vi "Read Action settings.vi"(8 "error in (no error)":errorcluster, 11 "Motor in":refnum<class "Motor.lvclass">) -> (0 "error out":errorcluster, 2 "Action settings":T1, 3 "Motor out":refnum<class "Motor.lvclass">)   [LabVIEW 2013, in "PowderDeposition.lvlib" / "Motor.lvclass"]
uses:
  Motor.lvclass
  Action-settings.ctl
  Motor.lvclass/Motor.ctl
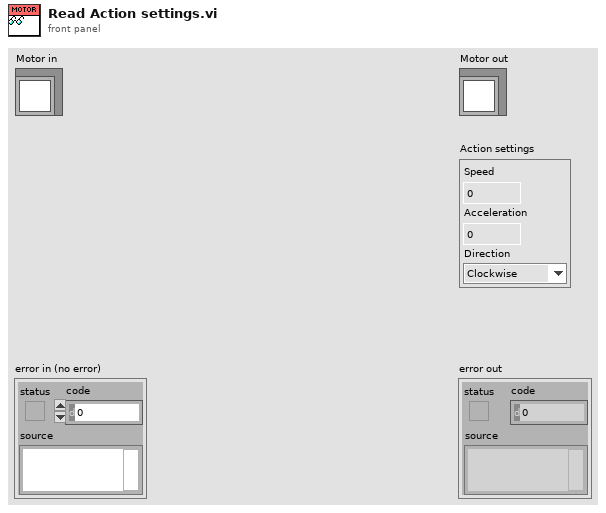
[diagram p1: front panel]
types:
  T1 = typedef "PowderDeposition.lvlib/Motor.lvclass/Action-settings.ctl" = cluster{"Speed":dbl, "Acceleration":dbl, "Direction":enum16{"Clockwise", "Counter-clockwise"}}
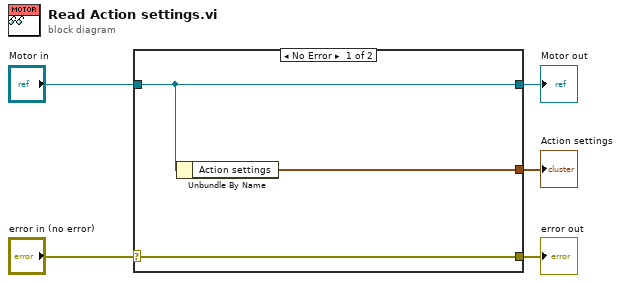
[diagram p0: block diagram]
diagram:
  n1 = case shown="No Error" "error in (no error)" {
    selector: "error in (no error)" -> [w8 w9]
    tunnel: [w8 w9] -> w4
    tunnel: [w7 w10] -> w2
    tunnel: "Motor in" -> [w7 w10]
    tunnel: [w6 _] -> w1
    frame No Error {
      n2 = Unbundle By Name(w7) -> ("Action settings"=w6:T1)
    }
    frame Error {
    }
  }
  "error out" <- w4
  "Motor out" <- w2
  "Action settings" <- w1
